vi "FunctionFromTag.vi"(8 "error in (no error)":errorcluster, 10 "MenuTag in":string, 11 "InsertFunctionMenu in":refnum<class "InsertFunctionMenu.lvclass">) -> (0 "error out":errorcluster, 2 "MenuItem out":string, 3 "InsertFunctionMenu out":refnum<class "InsertFunctionMenu.lvclass">)   [LabVIEW 2013, in "InsertFunctionMenu.lvclass"]
uses:
  InsertFunctionMenu.lvclass
  InsertFunctionMenu.lvclass/InsertFunctionMenu.ctl
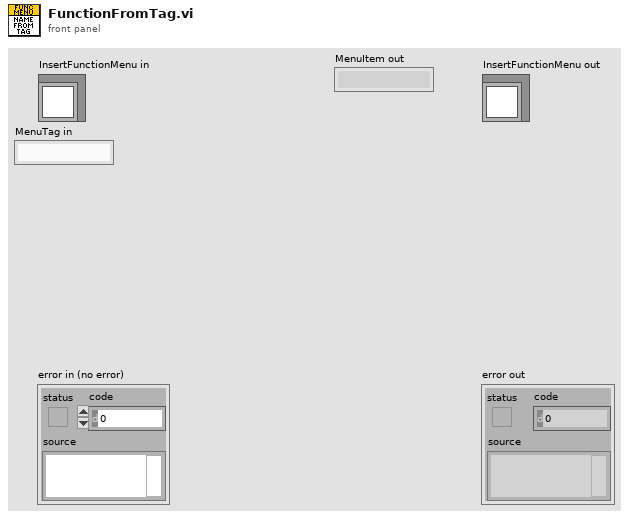
[diagram p1: front panel]
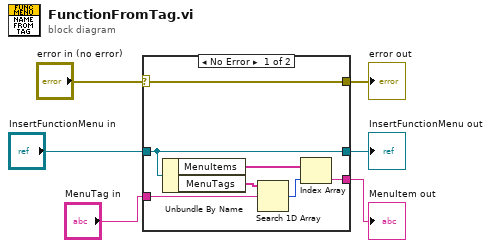
[diagram p0: block diagram]
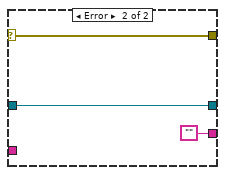
[diagram p2: hidden frame]
diagram:
  n1 = case shown="No Error" "error in (no error)" {
    selector: "error in (no error)" -> [w13 w16]
    tunnel: [w13 w16] -> w5
    tunnel: [w12 w15] -> w3
    tunnel: "InsertFunctionMenu in" -> [w12 w15]
    tunnel: "MenuTag in" -> [w10 _]
    tunnel: [w7 ""] -> w1
    frame No Error {
      n2 = Unbundle By Name(w12) -> ("MenuItems"=w8:string[], "MenuTags"=w11:string[])
      n3 = Search 1D Array(1D array=w11, element=w10) -> (index of element=w9:i32)  [unwired: 1 in]
      n4 = Index Array(array=w8, index=w9) -> (element=w7:string)
    }
    frame Error {
    }
  }
  "error out" <- w5
  "InsertFunctionMenu out" <- w3
  "MenuItem out" <- w1
